vi "Lift.vi"   [LabVIEW 2014]
uses:
  <vilib>/addons/control/pid/pid.llb/PID (DBL).vi
  <vilib>/addons/control/pid/NI_PID_pid.lvlib
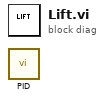
[diagram p0: block diagram]
diagram:
  n1 = call-poly <vilib>:"PID.vi"() -> ()  [unwired: 10 in, 2 out]
